vi "Write Setting 16bit.vi"(8 "error in (no error)":errorcluster, 9 "value":fxp<+,16,16>, 10 "FPGA Setting":T1, 11 "ScopeBase in":refnum<class "ScopeBase.lvclass">) -> (0 "error out":errorcluster, 3 "ScopeBase out":refnum<class "ScopeBase.lvclass">)   [LabVIEW 2013, in "ScopeBase.lvclass"]
uses:
  ScopeBase.lvclass
  FPGA/fpga_settings.ctl
  ScopeBase.lvclass/ScopeBase.ctl
  FpgaRef/FpgaRefBase/FpgaRefBase.lvclass
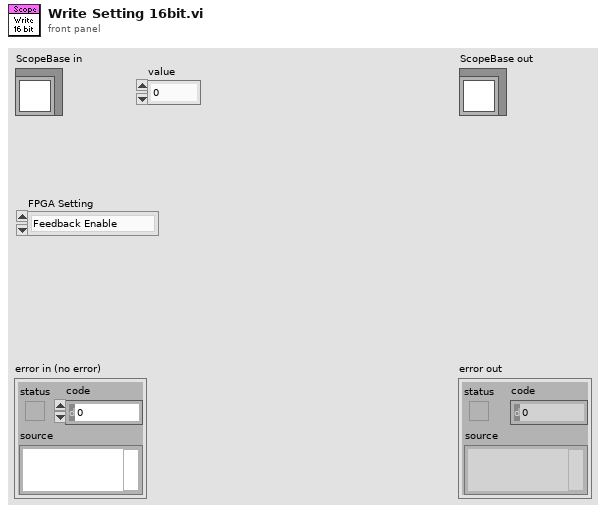
[diagram p1: front panel]
types:
  T1 = typedef "fpga_settings.ctl" = enum16{"Feedback Enable", "New FIR coeffs", "FIR shift", "Enable filter", "Set Downsample", "Downsample", "CIC Gain", "Record length", "Trigger samples", "Quiet time", "a_am", "b_am", "Use fixed delay", "fixed sin_fi", "fixed cos_fi", "Ki*Tau", "Kp", "Kd_Tau", "Fi_start", "Fi_delta", "DC_offs 0", "DC_offs 1", "DC_offs 2", "DC_offs 3", "Ki*Tau am", "Kp am", "Kd_Tau am", "Feedback AM", "Trigger delay", "Feedback delay", "Setpoint enable", "Beam enable", "Samples to acquire"}
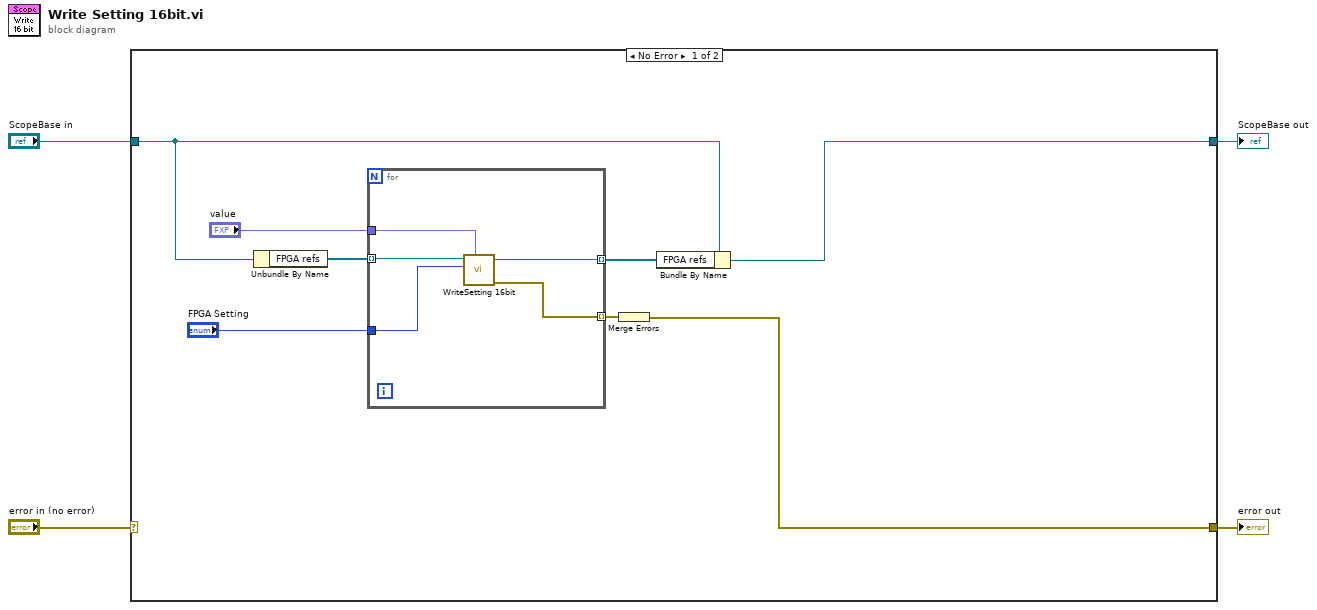
[diagram p0: block diagram]
diagram:
  n1 = case shown="No Error" "error in (no error)" {
    selector: "error in (no error)" -> [_ w19]
    tunnel: [w5 w19] -> w3
    tunnel: [w9 w18] -> w1
    tunnel: "ScopeBase in" -> [w10 w18]
    frame No Error {
      n2 = Unbundle By Name(w10) -> ("FPGA refs"=w12:refnum<class "FpgaRefBase.lvclass">[])
      n3 = for {
        tunnel: w12 -> [w17] mode=indexing
        tunnel: [w16] -> w11 mode=indexing
        tunnel: "value" -> [w15]
        tunnel: "FPGA Setting" -> [w14]
        tunnel: [w13] -> w6 mode=indexing
        n4 = call "WriteSetting 16bit.vi"("value"=w15, "FPGA Setting"=w14, "FpgaRefBase in"=w17) -> ("error out"=w13:errorcluster, "FpgaRefBase out"=w16:refnum<class "FpgaRefBase.lvclass">)  [unwired: 7 in]
      }
      n5 = Merge Errors(w6) -> (w5:errorcluster)
      n6 = Bundle By Name(cluster=w10, "FPGA refs"=w11) -> (w9:refnum<class "ScopeBase.lvclass">)
    }
    frame Error {
    }
  }
  "error out" <- w3
  "ScopeBase out" <- w1
